vi "Calculate Packet Cycles.vi"(10 "actual link data rate (B/s)":dbl, 11 "packet size":u32) -> (3 "packet cycles":u64)   [LabVIEW 2023, in "GettingStarted_Gen_148X_Host.lvlib"]
uses:
  GettingStarted_Gen_148X_Host.lvlib
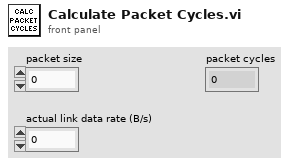
[diagram p1: front panel]
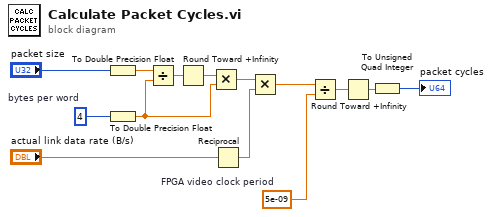
[diagram p0: block diagram]
diagram:
  w12 = 4  # bytes per word
  w4 = 5e-09  # FPGA video clock period
  n1 = To Double Precision Float(number="packet size") -> (double precision float=w11:dbl)
  n2 = To Double Precision Float(number=w12) -> (double precision float=w13:dbl)
  n3 = Divide(x=w11, y=w13) -> (x/y=w8:dbl)
  n4 = Round Toward +Infinity(x=w8) -> (ceil(x): smallest int >= x=w9:dbl)
  n5 = Multiply(x=w9, y=w13) -> (x*y=w14:dbl)
  n6 = Reciprocal(x="actual link data rate (B/s)") -> (1/x=w2:dbl)
  n7 = Multiply(x=w14, y=w2) -> (x*y=w3:dbl)
  n8 = Divide(x=w3, y=w4) -> (x/y=w5:dbl)
  n9 = Round Toward +Infinity(x=w5) -> (ceil(x): smallest int >= x=w6:dbl)
  n10 = To Unsigned Quad Integer(1:w6) -> (0:→"packet cycles":u64)
